vi "CAN Rx Q Ref Init.vi"(8 "error in (no error)":errorcluster) -> (0 "error out":errorcluster, 3 "CAN Read Q Out":T1)   [LabVIEW 2023, in "LTT_TeststandSteptypes.lvlib"]
uses:
  LTT_TeststandSteptypes.lvlib
  Control/CAN Read Q Ref.ctl
  <vilib>/xnet/xnet.llb/XNET Frame CAN.ctl
  <vilib>/xnet/xnet.llb/XNET Frame Type CAN.ctl
  Control/CAN FGV State.ctl
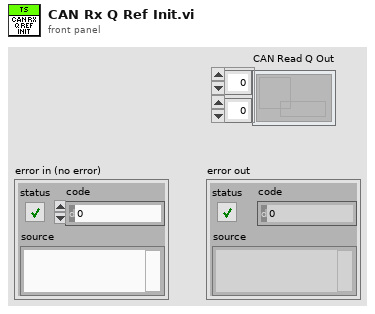
[diagram p1: front panel]
types:
  T1 = typedef "LTT_TeststandSteptypes.lvlib/CAN Read Q Ref.ctl" = refnum<queue>[][]
  T2 = typedef "LTT_TeststandSteptypes.lvlib/CAN FGV State.ctl" = enum16{"Init", "Get", "Set"}
  T3 = typedef "XNET Frame CAN.ctl" = cluster{"timestamp":timestamp, "payload":u8[], "identifier":u32, "type":T4, "extended?":bool, "echo?":bool}
  T4 = typedef "XNET Frame Type CAN.ctl" = u8
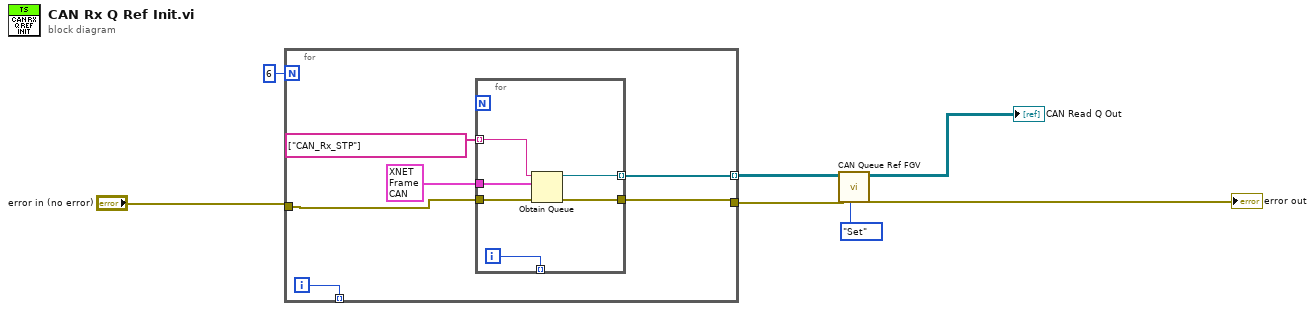
[diagram p0: block diagram]
diagram:
  n1 = for {
    N: 6 -> [_]
    tunnel: "error in (no error)" -> [w13]
    tunnel: [w10] -> w5 mode=indexing
    tunnel: [w9] -> _ mode=indexing
    tunnel: [w8] -> w6
    i -> [w9]
    n2 = for {
      tunnel: w13 -> [w19]
      tunnel: T3 {"timestamp"=timestamp(0 s since 1904-01-01), "payload"=[], "identifier"=0, "type"=0, "extended?"=FALSE, "echo?"=FALSE} ("CAN frame") -> [w18]
      tunnel: string[] ["CAN_Rx_STP"] -> [w17] mode=indexing
      tunnel: [w16] -> w10 mode=indexing
      tunnel: [w15] -> w8
      tunnel: [w14] -> _ mode=indexing
      i -> [w14]
      n3 = Obtain Queue(name (unnamed)=w17, element data type=w18, error in (no error)=w19) -> (queue out=w16:refnum<queue>, error out=w15:errorcluster)  [unwired: 2 in, 1 out]
    }
  }
  n4 = call "CAN Queue Ref FGV.vi"("CAN FGV State"=CAN_FGV_State."Set", "error in"=w6, "CAN Read Q In"=w5) -> ("error out"=→"error out":errorcluster, "CAN Read Q Out"=→"CAN Read Q Out":T1)  [unwired: 7 in]
